vi "Firstclick(debounce 2) 847v0(SubVI).vi"(1 "Input":bool) -> (0 "output":bool)   [LabVIEW 2012]
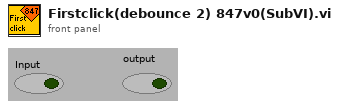
[diagram p1: front panel]
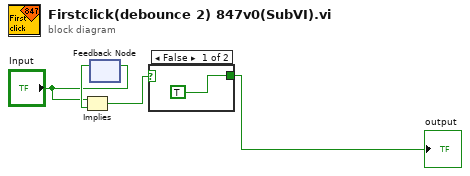
[diagram p0: block diagram]
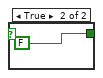
[diagram p2: hidden frame]
diagram:
  n1 = feedback-in #1("Input") -> ()
  n2 = feedback #1() -> (w3:bool)  [unwired: 1 in]
  n3 = Implies(1:w3, 2:"Input") -> (0:w4:bool)
  n4 = case shown="False" w4 {
    tunnel: [TRUE ("Boolean 2") FALSE ("Boolean 2")] -> w1
    frame False {
    }
    frame True {
    }
  }
  "output" <- w1
